vi "Comando movimiento micrometrico XY.vi"(0 "Activar movimiento en X":bool, 1 "VISA resource name":refnum<visa-resource-name>, 2 "Activar movimiento en Y":bool, 3 "Micras en X":dbl, 4 "error in":errorcluster, 5 "Micras en Y":dbl) -> (6 "Caso":i32, 7 "VISA resource name out":refnum<visa-resource-name>, 8 "error out":errorcluster)   [LabVIEW 2018]
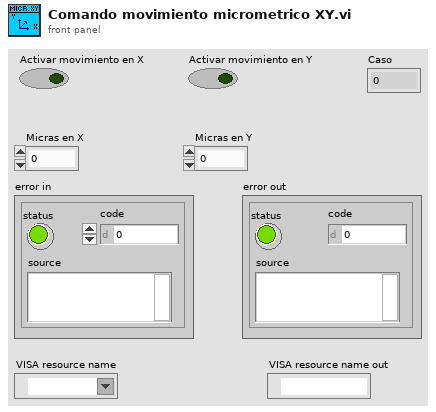
[diagram p1: front panel]
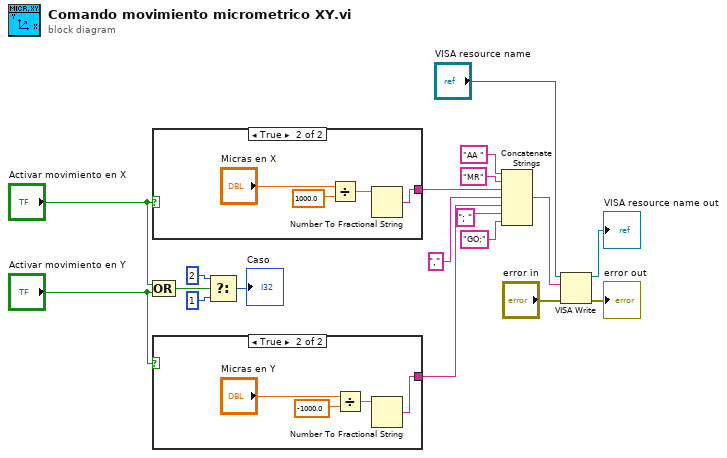
[diagram p0: block diagram]
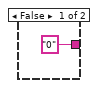
[diagram p2: hidden frame]
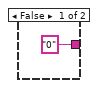
[diagram p3: hidden frame]
diagram:
  n1 = case shown="True" "Activar movimiento en X" {
    tunnel: ["0" w20] -> w12
    frame False {
    }
    frame True {
      n2 = Divide(x="Micras en X", y=1000.0) -> (x/y=w21:dbl)
      n3 = Number To Fractional String(number=w21) -> (F-format string=w20:string)  [unwired: 3 in]
    }
  }
  n4 = Compound Arithmetic op=OR("Activar movimiento en X", "Activar movimiento en Y") -> (w11:bool)
  n5 = case shown="True" "Activar movimiento en Y" {
    tunnel: ["0" ("String 2") w25] -> w13
    frame False {
    }
    frame True {
      n6 = Divide(x="Micras en Y", y=-1000.0) -> (x/y=w26:dbl)
      n7 = Number To Fractional String(number=w26) -> (F-format string=w25:string)  [unwired: 3 in]
    }
  }
  n8 = Select(t=2, s=w11, f=1) -> (s? t:f=→"Caso":i32)
  n9 = Concatenate Strings("AA " ("string"), "MR" ("string"), w12, "," ("string"), w13, "; " ("string"), "GO;" ("string")) -> (w1:string)
  n10 = VISA Write(VISA resource name="VISA resource name", write buffer=w1, error in (no error)="error in") -> (VISA resource name out=→"VISA resource name out":refnum<visa-resource-name>, error out=→"error out":errorcluster)  [unwired: 1 out]
